vi "LR-Select-process-steps.vi"(8 "error in (no error)":errorcluster, 11 "Laser characteristics":T2={"Zero level"=TRUE, "Stable level"=TRUE, "Reaction time"=TRUE, "Response time"=TRUE, "Stabilization time"=TRUE, "Shutdown time"=TRUE, "Extinction time"=TRUE, "Power spike"=TRUE}) -> (0 "error out":errorcluster, 2 "Steps":T1[](array[typedef]))   [LabVIEW 2013]
doc: "Use this template to build a VI to use as a subVI."
uses:
  Laser-characteristics.ctl
  TypeDefs/States.ctl
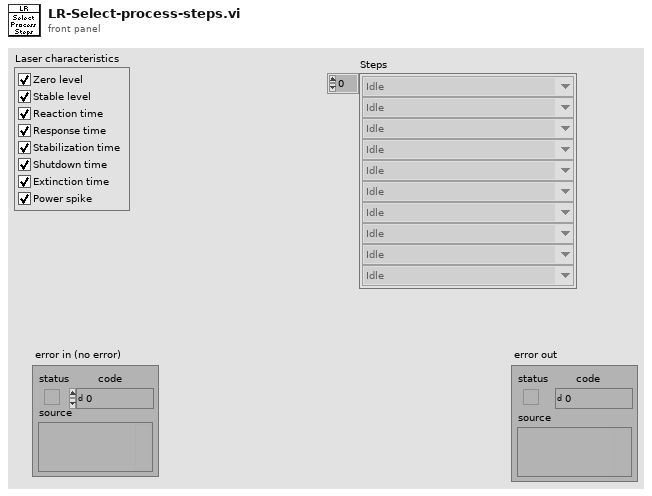
[diagram p1: front panel]
types:
  T1 = typedef "States.ctl" = enum16{"Initialize", "Idle", "Select files", "Edit characteristics", "Edit settings", "Start", "Load file", "Determine zero", "Determine stable level", "Divide samples", "Determine reaction time", "Determine response time", "Determine stabilization time", "Determine shutdown time", "Determine extinction time", "Detect spikes", "Display results", "Stop", "Pause", "Save", "Exit"}
  T2 = typedef "Laser-characteristics.ctl" = cluster{"Zero level":bool, "Stable level":bool, "Reaction time":bool, "Response time":bool, "Stabilization time":bool, "Shutdown time":bool, "Extinction time":bool, "Power spike":bool}
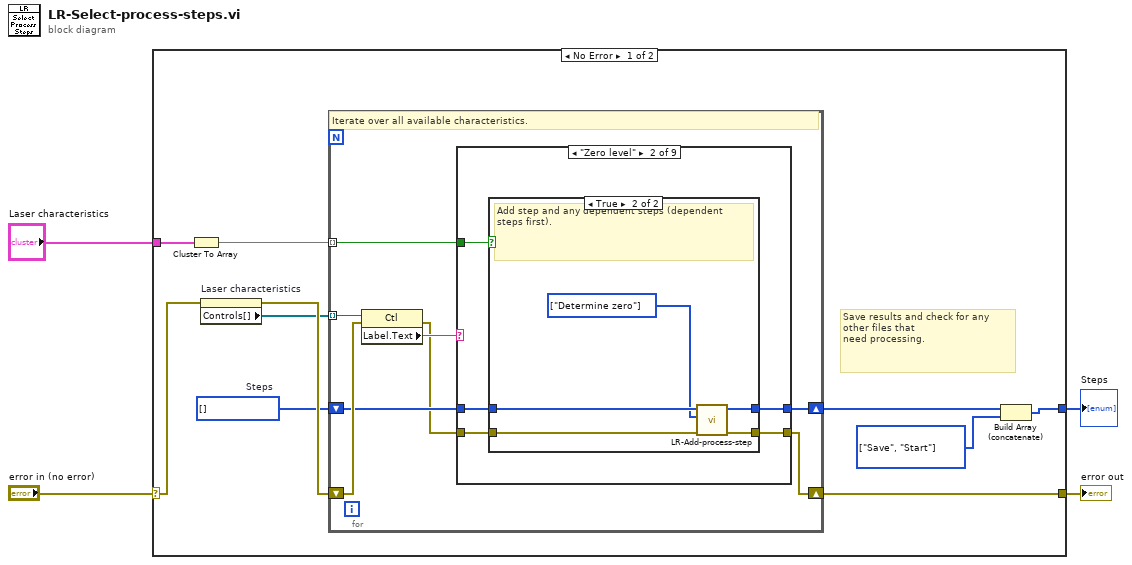
[diagram p0: block diagram]
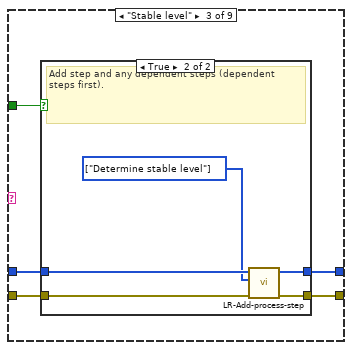
[diagram p4: hidden frame]
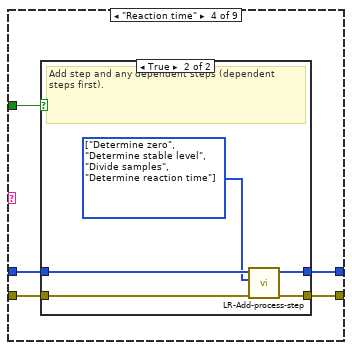
[diagram p6: hidden frame]
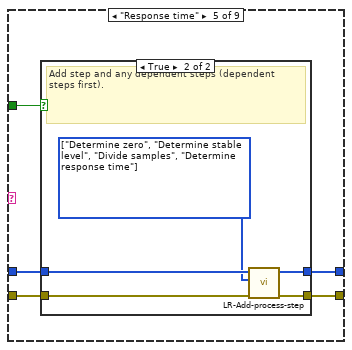
[diagram p8: hidden frame]
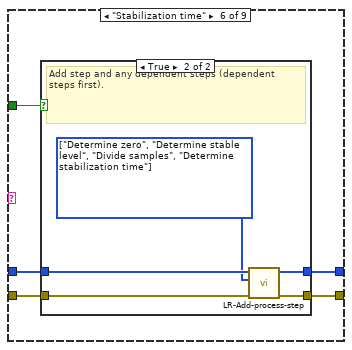
[diagram p10: hidden frame]
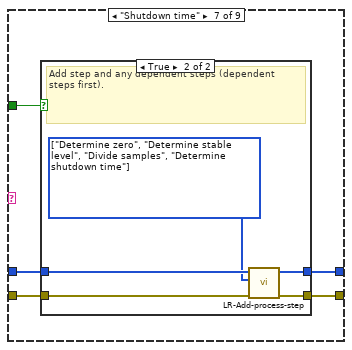
[diagram p12: hidden frame]
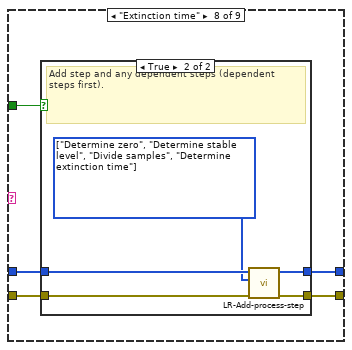
[diagram p14: hidden frame]
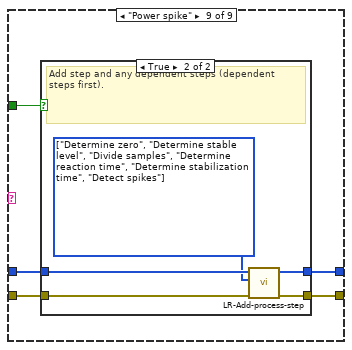
[diagram p16: hidden frame]
diagram:
  n1 = case shown="No Error" "error in (no error)" {
    selector: "error in (no error)" -> [w12 w121]
    tunnel: [w14 w121] -> w3
    tunnel: "Laser characteristics" -> [w13 _]
    tunnel: [w6 _] -> w1
    frame No Error {
      w5 = T1[] [enum."Save", enum."Start"] items=["Initialize", "Idle", "Select files", "Edit characteristics", "Edit settings", "Start", "Load file", "Determine zero", "Determine stable level", "Divide samples", "Determine reaction time", "Determine response time", "Determine stabilization time", "Determine shutdown time", "Determine extinction time", "Detect spikes", "Display results", "Stop", "Pause", "Save", "Exit"]
      w8 = T1[] [] items=["Initialize", "Idle", "Select files", "Edit characteristics", "Edit settings", "Start", "Load file", "Determine zero", "Determine stable level", "Divide samples", "Determine reaction time", "Determine response time", "Determine stabilization time", "Determine shutdown time", "Determine extinction time", "Detect spikes", "Display results", "Stop", "Pause", "Save", "Exit"]  # Steps
      # "Save results and check for any other files that \nneed processing."
      n2 = Cluster To Array(cluster=w13) -> (array=w9:bool[])
      n3 = property on="Laser characteristics" class="Clust (strict)"(error in=w12) -> (error out=w11:errorcluster, "Controls[]"=w10:refnum<vi>[])  [unwired: 1 in, 1 out]
      n4 = for {
        shift-right: [w15] -> w14
        shift-left: w11 -> [w21]
        tunnel: w10 -> [w22] mode=indexing
        tunnel: w9 -> [w19] mode=indexing
        shift-right: [w17] -> w7
        shift-left: w8 -> [w18]
        # "Iterate over all available characteristics."
        n5 = property class="Ctl"(reference=w22, error in=w21) -> (error out=w16:errorcluster, "Label.Text"=w20:string)  [unwired: 1 out]
        n6 = case shown="\"Zero level\"" w20 {
          tunnel: w19 -> [_ w29 w41 w53 w65 w77 w89 w101 w113]
          tunnel: w18 -> [w24 w28 w40 w52 w64 w76 w88 w100 w112]
          tunnel: [w24 w27 w39 w51 w63 w75 w87 w99 w111] -> w17
          tunnel: w16 -> [w23 w26 w38 w50 w62 w74 w86 w98 w110]
          tunnel: [w23 w25 w37 w49 w61 w73 w85 w97 w109] -> w15
          frame Default {
          }
          frame "Zero level" {
            n7 = case shown="True" w29 {
              tunnel: w28 -> [w31 w36]
              tunnel: [w31 w35] -> w27
              tunnel: w26 -> [w30 w33]
              tunnel: [w30 w32] -> w25
              frame False {
                # "Characteristic not used, do not add it to the process steps."
              }
              frame True {
                w34 = T1[] [enum."Determine zero"] items=["Initialize", "Idle", "Select files", "Edit characteristics", "Edit settings", "Start", "Load file", "Determine zero", "Determine stable level", "Divide samples", "Determine reaction time", "Determine response time", "Determine stabilization time", "Determine shutdown time", "Determine extinction time", "Detect spikes", "Display results", "Stop", "Pause", "Save", "Exit"]
                # "Add step and any dependent steps (dependent steps first)."
                n8 = call "LR-Add-process-step.vi"("error in (no error)"=w33, "Steps to add"=w34, "Current steps in"=w36) -> ("error out"=w32:errorcluster, "Current steps"=w35:T1[])  [unwired: 7 in]
              }
            }
          }
          frame "Stable level" {
            n9 = case shown="True" w41 {
              tunnel: w40 -> [w43 w48]
              tunnel: [w43 w47] -> w39
              tunnel: w38 -> [w42 w45]
              tunnel: [w42 w44] -> w37
              frame False {
                # "Characteristic not used, do not add it to the process steps."
              }
              frame True {
                w46 = T1[] [enum."Determine stable level"] items=["Initialize", "Idle", "Select files", "Edit characteristics", "Edit settings", "Start", "Load file", "Determine zero", "Determine stable level", "Divide samples", "Determine reaction time", "Determine response time", "Determine stabilization time", "Determine shutdown time", "Determine extinction time", "Detect spikes", "Display results", "Stop", "Pause", "Save", "Exit"]
                # "Add step and any dependent steps (dependent steps first)."
                n10 = call "LR-Add-process-step.vi"("error in (no error)"=w45, "Steps to add"=w46, "Current steps in"=w48) -> ("error out"=w44:errorcluster, "Current steps"=w47:T1[])  [unwired: 7 in]
              }
            }
          }
          frame "Reaction time" {
            n11 = case shown="True" w53 {
              tunnel: w52 -> [w55 w60]
              tunnel: [w55 w59] -> w51
              tunnel: w50 -> [w54 w57]
              tunnel: [w54 w56] -> w49
              frame False {
                # "Characteristic not used, do not add it to the process steps."
              }
              frame True {
                w58 = T1[] [enum."Determine zero", enum."Determine stable level", enum."Divide samples", enum."Determine reaction time"] items=["Initialize", "Idle", "Select files", "Edit characteristics", "Edit settings", "Start", "Load file", "Determine zero", "Determine stable level", "Divide samples", "Determine reaction time", "Determine response time", "Determine stabilization time", "Determine shutdown time", "Determine extinction time", "Detect spikes", "Display results", "Stop", "Pause", "Save", "Exit"]
                # "Add step and any dependent steps (dependent steps first)."
                n12 = call "LR-Add-process-step.vi"("error in (no error)"=w57, "Steps to add"=w58, "Current steps in"=w60) -> ("error out"=w56:errorcluster, "Current steps"=w59:T1[])  [unwired: 7 in]
              }
            }
          }
          frame "Response time" {
            n13 = case shown="True" w65 {
              tunnel: w64 -> [w67 w72]
              tunnel: [w67 w71] -> w63
              tunnel: w62 -> [w66 w69]
              tunnel: [w66 w68] -> w61
              frame False {
                # "Characteristic not used, do not add it to the process steps."
              }
              frame True {
                w70 = T1[] [enum."Determine zero", enum."Determine stable level", enum."Divide samples", enum."Determine response time"] items=["Initialize", "Idle", "Select files", "Edit characteristics", "Edit settings", "Start", "Load file", "Determine zero", "Determine stable level", "Divide samples", "Determine reaction time", "Determine response time", "Determine stabilization time", "Determine shutdown time", "Determine extinction time", "Detect spikes", "Display results", "Stop", "Pause", "Save", "Exit"]
                # "Add step and any dependent steps (dependent steps first)."
                n14 = call "LR-Add-process-step.vi"("error in (no error)"=w69, "Steps to add"=w70, "Current steps in"=w72) -> ("error out"=w68:errorcluster, "Current steps"=w71:T1[])  [unwired: 7 in]
              }
            }
          }
          frame "Stabilization time" {
            n15 = case shown="True" w77 {
              tunnel: w76 -> [w79 w84]
              tunnel: [w79 w83] -> w75
              tunnel: w74 -> [w78 w81]
              tunnel: [w78 w80] -> w73
              frame False {
                # "Characteristic not used, do not add it to the process steps."
              }
              frame True {
                w82 = T1[] [enum."Determine zero", enum."Determine stable level", enum."Divide samples", enum."Determine stabilization time"] items=["Initialize", "Idle", "Select files", "Edit characteristics", "Edit settings", "Start", "Load file", "Determine zero", "Determine stable level", "Divide samples", "Determine reaction time", "Determine response time", "Determine stabilization time", "Determine shutdown time", "Determine extinction time", "Detect spikes", "Display results", "Stop", "Pause", "Save", "Exit"]
                # "Add step and any dependent steps (dependent steps first)."
                n16 = call "LR-Add-process-step.vi"("error in (no error)"=w81, "Steps to add"=w82, "Current steps in"=w84) -> ("error out"=w80:errorcluster, "Current steps"=w83:T1[])  [unwired: 7 in]
              }
            }
          }
          frame "Shutdown time" {
            n17 = case shown="True" w89 {
              tunnel: w88 -> [w91 w96]
              tunnel: [w91 w95] -> w87
              tunnel: w86 -> [w90 w93]
              tunnel: [w90 w92] -> w85
              frame False {
                # "Characteristic not used, do not add it to the process steps."
              }
              frame True {
                w94 = T1[] [enum."Determine zero", enum."Determine stable level", enum."Divide samples", enum."Determine shutdown time"] items=["Initialize", "Idle", "Select files", "Edit characteristics", "Edit settings", "Start", "Load file", "Determine zero", "Determine stable level", "Divide samples", "Determine reaction time", "Determine response time", "Determine stabilization time", "Determine shutdown time", "Determine extinction time", "Detect spikes", "Display results", "Stop", "Pause", "Save", "Exit"]
                # "Add step and any dependent steps (dependent steps first)."
                n18 = call "LR-Add-process-step.vi"("error in (no error)"=w93, "Steps to add"=w94, "Current steps in"=w96) -> ("error out"=w92:errorcluster, "Current steps"=w95:T1[])  [unwired: 7 in]
              }
            }
          }
          frame "Extinction time" {
            n19 = case shown="True" w101 {
              tunnel: w100 -> [w103 w108]
              tunnel: [w103 w107] -> w99
              tunnel: w98 -> [w102 w105]
              tunnel: [w102 w104] -> w97
              frame False {
                # "Characteristic not used, do not add it to the process steps."
              }
              frame True {
                w106 = T1[] [enum."Determine zero", enum."Determine stable level", enum."Divide samples", enum."Determine extinction time"] items=["Initialize", "Idle", "Select files", "Edit characteristics", "Edit settings", "Start", "Load file", "Determine zero", "Determine stable level", "Divide samples", "Determine reaction time", "Determine response time", "Determine stabilization time", "Determine shutdown time", "Determine extinction time", "Detect spikes", "Display results", "Stop", "Pause", "Save", "Exit"]
                # "Add step and any dependent steps (dependent steps first)."
                n20 = call "LR-Add-process-step.vi"("error in (no error)"=w105, "Steps to add"=w106, "Current steps in"=w108) -> ("error out"=w104:errorcluster, "Current steps"=w107:T1[])  [unwired: 7 in]
              }
            }
          }
          frame "Power spike" {
            n21 = case shown="True" w113 {
              tunnel: w112 -> [w115 w120]
              tunnel: [w115 w119] -> w111
              tunnel: w110 -> [w114 w117]
              tunnel: [w114 w116] -> w109
              frame False {
                # "Characteristic not used, do not add it to the process steps."
              }
              frame True {
                w118 = T1[] [enum."Determine zero", enum."Determine stable level", enum."Divide samples", enum."Determine reaction time", enum."Determine stabilization time", enum."Detect spikes"] items=["Initialize", "Idle", "Select files", "Edit characteristics", "Edit settings", "Start", "Load file", "Determine zero", "Determine stable level", "Divide samples", "Determine reaction time", "Determine response time", "Determine stabilization time", "Determine shutdown time", "Determine extinction time", "Detect spikes", "Display results", "Stop", "Pause", "Save", "Exit"]
                # "Add step and any dependent steps (dependent steps first)."
                n22 = call "LR-Add-process-step.vi"("error in (no error)"=w117, "Steps to add"=w118, "Current steps in"=w120) -> ("error out"=w116:errorcluster, "Current steps"=w119:T1[])  [unwired: 7 in]
              }
            }
          }
        }
      }
      n23 = Build Array (concatenate)(w7, w5) -> (w6:T1[])
    }
    frame Error {
    }
  }
  "error out" <- w3
  "Steps" <- w1
